vi "Helper - ToggleOverrides.vi"(4 "Map Mode Tab Control Ref":refnum<vi>, 6 "OCU Tab Control Ref":refnum<vi>, 7 "FocusObj":refnum<vi>, 8 "Rudder Override?":bool, 9 "Sail Override?":bool, 10 "VKey":T1=enum."Up", 11 "Char":i16) -> (1 "Override Rudder":bool, 2 "Override Sail":bool)   [LabVIEW 2011]
doc: "Takes in current values of sail and rudder override and togges them if the correct button is hit.\nOnly does something if you're actually looking at the OCU - use the event structure to get FocusObj.\n\nPotential problem: if you hit the button on the OCU and the keyboard button at the same time, they might end up cancelling each other out.... But, then again, why would you do that?\n\n-Elizabeth Mahon"
uses:
  <vilib>/event_ctls.llb/eventvkey.ctl
panel:
  out "*(type *) &x":string
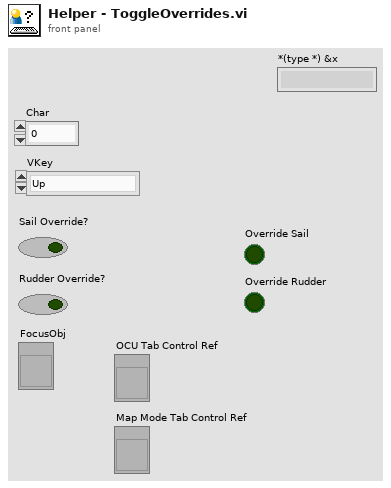
[diagram p1: front panel]
types:
  T1 = typedef "eventvkey.ctl" = enum16{"ASCII", "Enter", "Return", "Shift", "Ctrl", "Alt", "Cmd", "Opt", "Caps", "NumLock", "Clear", "Break", "Up", "Down", "Left", "Right", "Insert", "Delete", "Home", "End", "PageUp", "PageDown", "Escape", "Help", "Pause", "ScrollLock", "F1", "F2", "F3", "F4", "F5", "F6", "F7", "F8", "F9", "F10", "F11", "F12", "F13", "F14", "F15", "F16", "F17", "F18", "F19", "F20", "F21", "F22", "F23", "F24", "Play", "VolumeUp", "VolumeDown", "Mute", "Two Byte Char"}
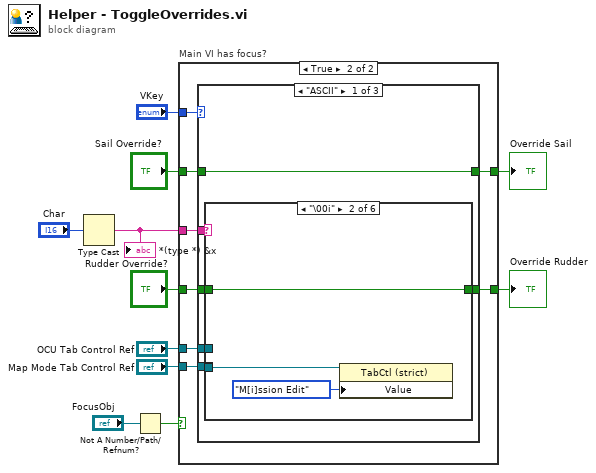
[diagram p0: block diagram]
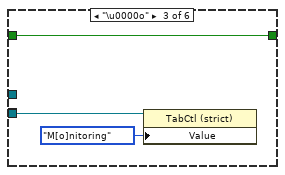
[diagram p4: hidden frame]
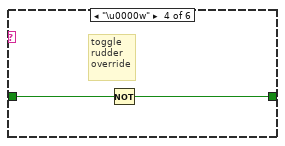
[diagram p5: hidden frame]
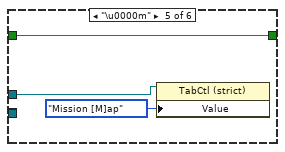
[diagram p6: hidden frame]
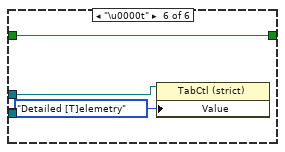
[diagram p7: hidden frame]
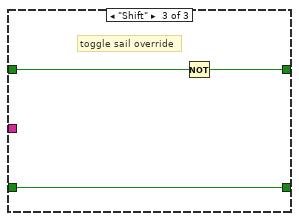
[diagram p9: hidden frame]
diagram:
  n1 = Type Cast(x="Char") -> (*(type *) &x=w3:string)  [unwired: 1 in]
  "*(type *) &x" <- w3
  n2 = Not A Number/Path/Refnum?(number/path/refnum="FocusObj") -> (NaN/Path/Refnum?=w9:bool)
  n3 = case "Main VI has focus?" shown="True" w9 {
    tunnel: "VKey" -> [_ w21]
    tunnel: "Sail Override?" -> [w13 w20]
    tunnel: [w13 w19] -> w7
    tunnel: "Rudder Override?" -> [w12 w18]
    tunnel: [w12 w17] -> w5
    tunnel: w3 -> [_ w16]
    tunnel: "OCU Tab Control Ref" -> [_ w15]
    tunnel: "Map Mode Tab Control Ref" -> [_ w14]
    frame False {
    }
    frame True {
      n4 = case shown="\"ASCII\"" w21 {
        tunnel: w20 -> [w27 w44 w46]
        tunnel: [w27 w44 w47] -> w19
        tunnel: w18 -> [w26 w43 w45]
        tunnel: [w25 w43 w45] -> w17
        tunnel: w16 -> [w24 _ _]
        tunnel: w15 -> [w23 _ _]
        tunnel: w14 -> [w22 _ _]
        frame "ASCII" {
          n5 = case shown="\"\\00i\"" w24 {
            tunnel: w26 -> [w28 w31 w34 w36 w39 w42]
            tunnel: [w28 w31 w34 w35 w39 w42] -> w25
            tunnel: w23 -> [_ _ _ _ w37 w40]
            tunnel: w22 -> [_ _ _ _ _ _]
            tunnel: w22 -> [_ w30 w33 _ _ _]
            frame Default {
            }
            frame "\u0000i" {
              n6 = property class="TabCtl (strict)"(reference=w30, "Value"=enum32{"M[i]ssion Edit", "M[o]nitoring"}."M[i]ssion Edit") -> ()  [unwired: 1 in, 2 out]
            }
            frame "\u0000o" {
              n7 = property class="TabCtl (strict)"(reference=w33, "Value"=enum32{"M[i]ssion Edit", "M[o]nitoring"}."M[o]nitoring") -> ()  [unwired: 1 in, 2 out]
            }
            frame "\u0000w" {
              # "toggle\nrudder\noverride"
              n8 = Not(x=w36) -> (.not. x?=w35:bool)
            }
            frame "\u0000m" {
              n9 = property class="TabCtl (strict)"(reference=w37, "Value"=enum32{"Mission [M]ap", "Detailed [T]elemetry"}."Mission [M]ap") -> ()  [unwired: 1 in, 2 out]
            }
            frame "\u0000t" {
              n10 = property class="TabCtl (strict)"(reference=w40, "Value"=enum32{"Mission [M]ap", "Detailed [T]elemetry"}."Detailed [T]elemetry") -> ()  [unwired: 1 in, 2 out]
            }
          }
        }
        frame Default {
        }
        frame "Shift" {
          # "toggle sail override"
          n11 = Not(x=w46) -> (.not. x?=w47:bool)
        }
      }
    }
  }
  "Override Sail" <- w7
  "Override Rudder" <- w5
